vi "PH_PILS.PC _SwitchKnob.vi"(0 "i ref in":refnum<vi>, 2 "serviceName":string, 3 "Value":i32, 5 "error IO":errorcluster) -> (14 "i ref out":refnum<vi>, 19 "error out":errorcluster)   [LabVIEW 2014, in "PH_PILS.lvlib"]
uses:
  PH_PILS.lvlib
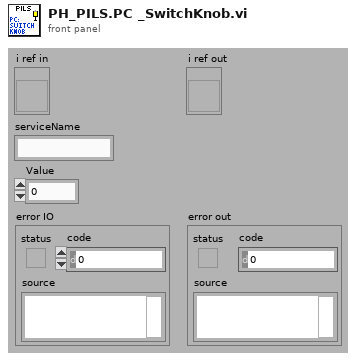
[diagram p1: front panel]
types:
  T1 = typedef "PH_PILS.lvlib/PH_PILS.i attribute.ctl" = cluster{"Boolean":cluster{"GUI Ref":refnum<vi>, "Status":i32}[], "GUI Refs Exp. Shutters":cluster{"1":refnum<vi>, "2":refnum<vi>, "3":refnum<vi>, "4":refnum<vi>}, "Tristate2Run GUI Refs":refnum<vi>[], "EO-Likes":cluster{"GUI Ref":refnum<vi>, "Status":i32}[], "Operation Mode":cluster{"Operation Mode":T2, "GUI":cluster{"Ref State":refnum<vi>, "Ref":refnum<vi>}, "Servicemode":cluster{"Tagname":string, "Status":i32}, "Labormode":cluster{"Tagname":string, "Status":i32}, "Searchmode":cluster{"Tagname":string, "Status":i32}, "Shotmode":cluster{"Tagname":string, "Status":i32}}, "Submode":cluster{"Submode":T3, "GUI":cluster{"Ref State":refnum<vi>, "Ref":refnum<vi>}, "Submode":cluster{"Tagname":string, "Status":i32}}, "Experiment":cluster{"Experiment":enum16{"unknown", "intern", "4 (Z6)", "3", "2", "1"}, "GUI":cluster{"Ref State":refnum<vi>, "Ref":refnum<vi>}, "intern":cluster{"Tagname":string, "Status":i32}, "Exp 4":cluster{"Tagname":string, "Status":i32}, "Exp 3":cluster{"Tagname":string, "Status":i32}, "Exp 2":cluster{"Tagname":string, "Status":i32}, "Exp 1":cluster{"Tagname":string, "Status":i32}}, "TristateNormal":cluster{"GUI Ref":refnum<vi>, "Status":i32}[], "Door Tags":cluster{"GUI Ref":refnum<vi>, "Status":i32}[], "GUIlessTags":cluster{"Name":string, "Status":i32}[], "Beamline GUI Refs":refnum<vi>[], "Special Boolean":cluster{"GUI Ref":refnum<vi>, "Status":i32}[], "Laserpower":cluster{"GUI Ref":refnum<vi>, "Status":i32}[], "Shutter":cluster{"GUI Ref":refnum<vi>, "Status":i32}[], "Tristate EO Like":cluster{"GUI Ref":refnum<vi>, "Status":i32}[], "PP":cluster{"GUI Ref":refnum<vi>, "Status":i32, "Head Ref":refnum<vi>, "Slider Ref":refnum<vi>}[], "Switch Knobs":cluster{"GUI Ref":refnum<vi>, "Status":i32}[], "Latch Knob GUI Refs":refnum<vi>[], "FailureCounter":i32, "Enabled Status":cluster{"Laser":i32, "PreAmp":i32, "MainAmp":i32}, "Mercury":refnum<vi>, "Instance Rods":string, "Logfile":path, "Beckhoff-Instance Internal":string, "Beckhoff-Instance External":string, "Enabling Rights":cluster{"Name":string, "Password":string, "PA?":bool, "MA?":bool, "Exp?":bool}[]}
  T2 = typedef "PH_PILS.lvlib/PH_PILS.Operation Mode.ctl" = enum16{"unknown", "Service", "Labor", "Search", "Shot"}
  T3 = typedef "PH_PILS.lvlib/PH_PILS.Submode.ctl" = enum16{"unknown", "HV-Normal", "HV-Test"}
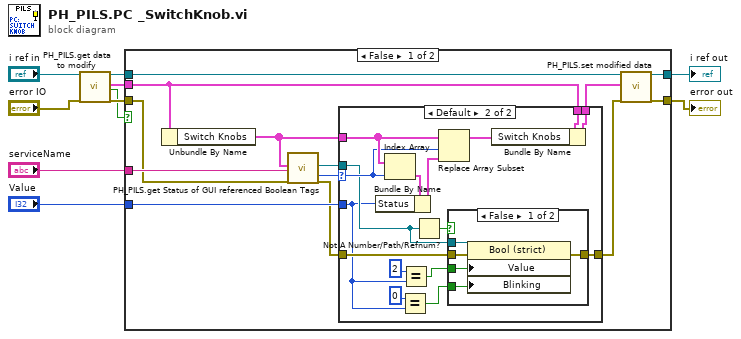
[diagram p0: block diagram]
diagram:
  n1 = call "PH_PILS.get data to modify.vi"("i ref in"="i ref in", "error in (no error)"="error IO") -> ("i ref out"=w4:refnum<vi>, "i attribute"=w5:T1, "timed out"=w1:bool, "error out"=w6:errorcluster)  [unwired: 14 in]
  n2 = case shown="False" w1 {
    tunnel: "Value" -> [w18 _]
    tunnel: "serviceName" -> [w16 _]
    tunnel: w6 -> [w14 w48]
    tunnel: w5 -> [w20 _]
    tunnel: w4 -> [w23 w49]
    tunnel: [w22 w49] -> w3
    tunnel: [w21 w48] -> w2
    frame False {
      n3 = Unbundle By Name(w20) -> ("Switch Knobs"=w17:cluster{"GUI Ref":refnum<vi>, "Status":i32}[])
      n4 = call "PH_PILS.get Status of GUI referenced Boolean Tags.vi"("Tags"=w17, "Tagname"=w16, "error in"=w14) -> ("GUI Ref"=w11:refnum<vi>, "index of element"=w15:i32, "error out"=w13:errorcluster)  [unwired: 13 in, 1 out]
      n5 = case shown="Default" w15 {
        selector: w15 -> [_ w35]
        tunnel: w17 -> [_ w41]
        tunnel: w20 -> [w25 w40]
        tunnel: [w25 w39] -> w19
        tunnel: w18 -> [_ w26]
        tunnel: w13 -> [w24 w33]
        tunnel: [w24 w32] -> w12
        tunnel: w11 -> [_ w29]
        frame -1 {
        }
        frame Default {
          n6 = Index Array(array=w41, index=w35) -> (element=w37:cluster{"GUI Ref":refnum<vi>, "Status":i32})
          n7 = Bundle By Name(cluster=w37, "Status"=w26) -> (w36:cluster{"GUI Ref":refnum<vi>, "Status":i32})
          n8 = Equal?(x=0, y=w26) -> (x = y?=w27:bool)
          n9 = Equal?(x=2, y=w26) -> (x = y?=w28:bool)
          n10 = Not A Number/Path/Refnum?(number/path/refnum=w29) -> (NaN/Path/Refnum?=w34:bool)
          n11 = Replace Array Subset(array=w41, new element=w36, index=w35) -> (w38:cluster{"GUI Ref":refnum<vi>, "Status":i32}[])
          n12 = case shown="False" w34 {
            tunnel: w29 -> [w46 _]
            tunnel: w28 -> [w45 _]
            tunnel: w33 -> [w44 w47]
            tunnel: [w43 w47] -> w32
            tunnel: w27 -> [w42 _]
            frame False {
              n13 = property class="Bool (strict)"(reference=w46, error in=w44, "Value"=w45, "Blinking"=w42) -> (error out=w43:errorcluster)  [unwired: 1 out]
            }
            frame True {
            }
          }
          n14 = Bundle By Name(cluster=w40, "Switch Knobs"=w38) -> (w39:T1)
        }
      }
      n15 = call "PH_PILS.set modified data.vi"("i ref in"=w23, "i attribute"=w19, "error in (no error)"=w12) -> ("i ref out"=w22:refnum<vi>, "error out"=w21:errorcluster)  [unwired: 15 in]
    }
    frame True {
    }
  }
  "error out" <- w2
  "i ref out" <- w3
